vi "Host Send to PXI.vi"(8 "Messages":T1, 11 "endpoint in":refnum<k21>) -> (3 "endpoint out":refnum<k21>)   [LabVIEW 2018]
uses:
  Host Messages.ctl
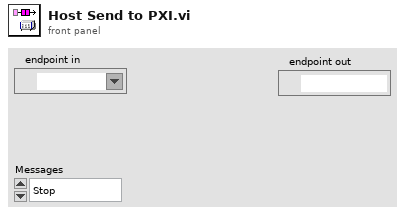
[diagram p1: front panel]
types:
  T1 = typedef "Host Messages.ctl" = enum16{"Stop", "Log Data", "Confirm File Name"}
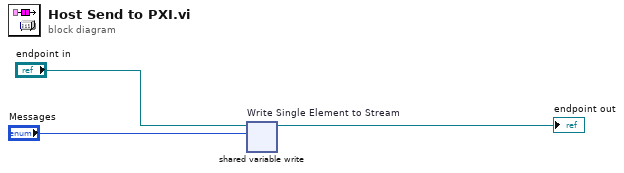
[diagram p0: block diagram]
diagram:
  n1 = shared-variable-write "Write Single Element to Stream"("endpoint in", "Messages") -> (→"endpoint out":refnum<k21>)  [unwired: 2 in, 2 out]
